vi "DefaultPsTactic.vi"(8 "error in (no error)":errorcluster, 9 "Game in":refnum<class "Game.lvclass">, 10 "Robot":refnum<class "Robot.lvclass">, 11 "DefaultPsTactic in":refnum<class "DefaultPsTactic.lvclass">) -> (0 "error out":errorcluster, 2 "Robot out":refnum<class "Robot.lvclass">, 3 "DefaultPsTactic out":refnum<class "DefaultPsTactic.lvclass">)   [LabVIEW 2018, in "DefaultPsTactic.lvclass"]
uses:
  DefaultPsTactic.lvclass
  C:/Users/anton/Desktop/roboime/PS 2020.1/SSL_AI/Tactic_class/Tactic.lvclass
  Robot_class/Robot.lvclass
  Game_class/Game.lvclass
  Tactic_class/Tactic.lvclass/Tactic.ctl
  TestTactic_class/States.ctl
  Robot_class/tactics.ctl
  Robot_class/Robot.lvclass/Robot.ctl
  Tactic_class/Read Skillbook.vi
  Robot_class/Write tactic.vi
  Skillbook_class/Skillbook.lvclass
  AttackPsSkill_class/AttackPsSkill.lvclass
  DefensePsSkill_class/DefensePsSkill.lvclass
panel:
  out "x .or. y?":bool
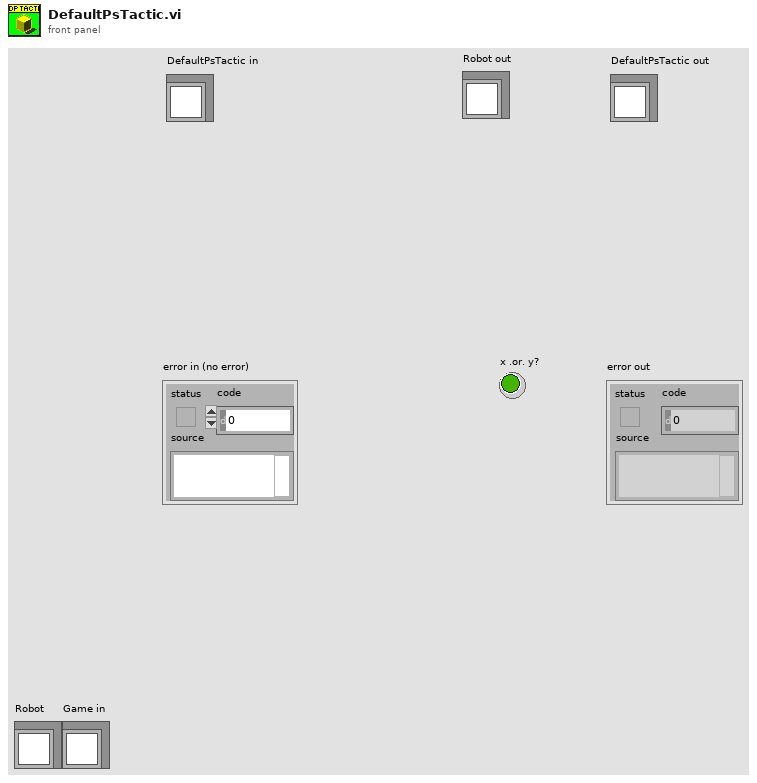
[diagram p1: front panel]
types:
  T1 = typedef "tactics.ctl" = enum16{"PenaltyAttacker", "DefaultPs", "PassObserver", "PenaltyDefense", "Test", "DefendGoal", "Marker", "FollowAttacker", "DefendArea", "Shoot", "AttackerAimGoal", "AttackerBallOutOfField", "AttackerBlock", "AttackerStop", "Duelist", "Halt", "ZigZag", "GoTo", "Timeout", "KickToPassReceiver", "PositionToReceivePass", "PassReceiver", "WaitPass"}
  T2 = typedef "States.ctl" = enum16{"Exit", "AttackPs", "DefensePs"}
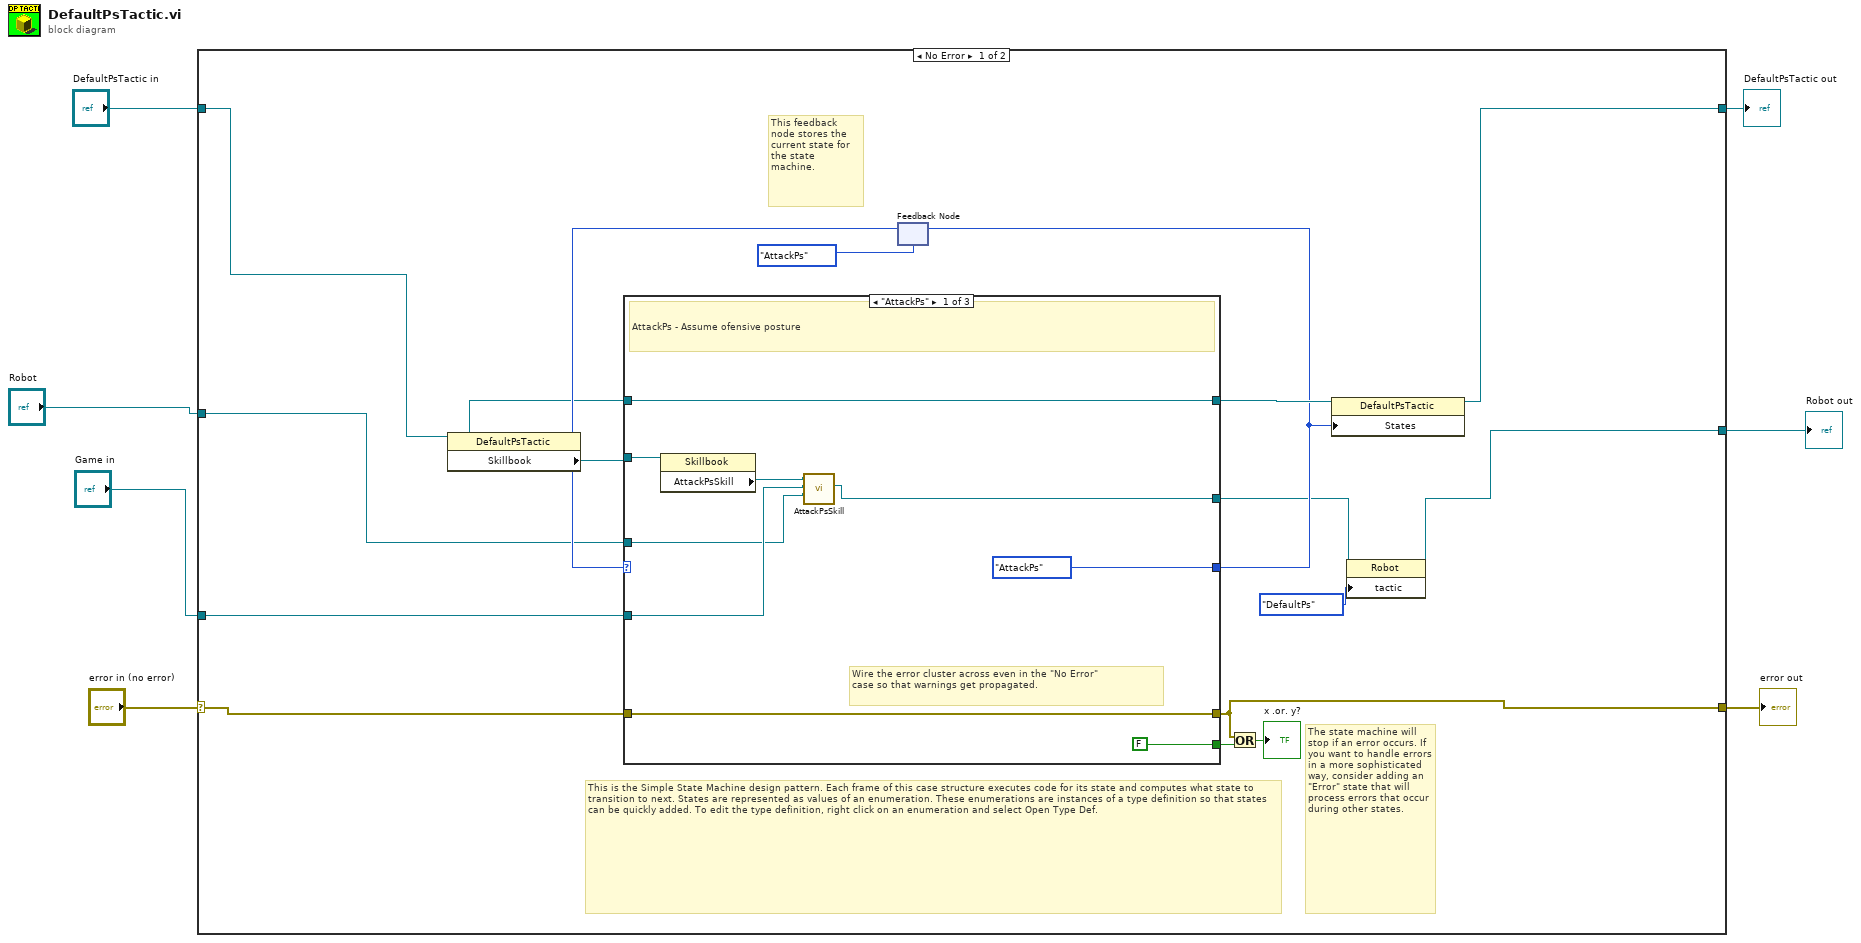
[diagram p0: block diagram]
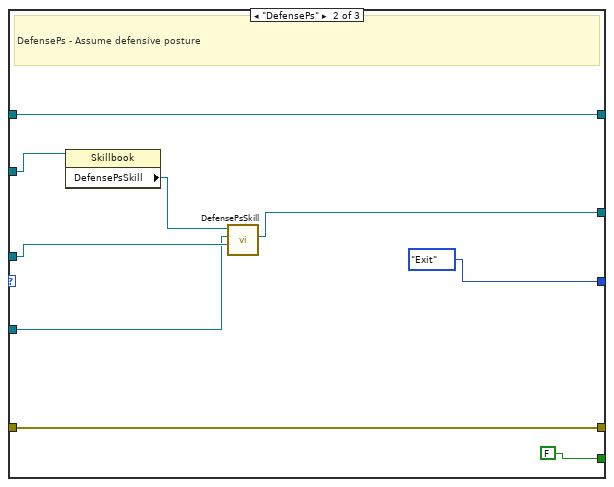
[diagram p2: hidden frame]
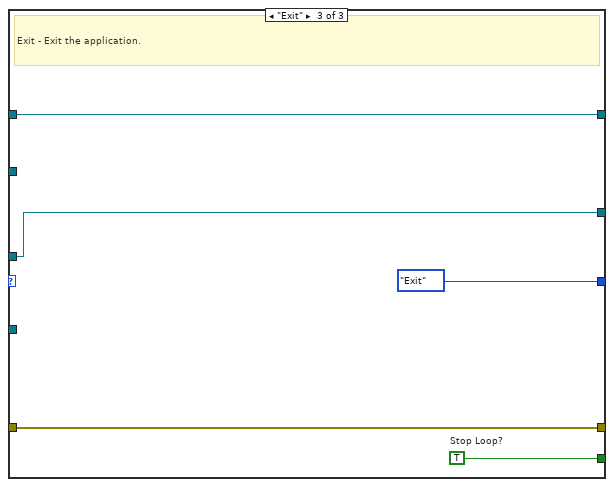
[diagram p3: hidden frame]
diagram:
  n1 = case shown="No Error" "error in (no error)" {
    selector: "error in (no error)" -> [w10 w48]
    tunnel: [w9 w48] -> w6
    tunnel: [w13 w47] -> w4
    tunnel: "DefaultPsTactic in" -> [w14 w47]
    tunnel: "Robot" -> [w12 _]
    tunnel: "Game in" -> [w11 _]
    tunnel: [w8 _] -> w1
    frame No Error {
      # "The state machine will stop if an error occurs. If you want to handle errors in a more sophisticated way, consider adding an \"Error\" state that will process errors that occur during other states."
      # "This feedback node stores the current state for the state machine."
      # "This is the Simple State Machine design pattern. Each frame of this case structure executes code for its state and computes what state to transition to next. States are represented as values of an enumeration. These enumerations are instances of a type definition so that states can be quickly added. To edit the type definition, right click on an enumeration and select Open Type Def."
      # "Wire the error cluster across even in the \"No Error\"\ncase so that warnings get propagated."
      n2 = property class="DefaultPsTactic"(reference=w14) -> ("Skillbook"=w19:refnum<class "Skillbook.lvclass">)  [unwired: 1 in, 2 out]
      n3 = feedback #1(States."AttackPs" ("States")) -> (w21:T2)
      n4 = case shown="\"AttackPs\"" w21 {
        tunnel: [States."AttackPs" ("States") States."Exit" ("States") States."Exit" ("States")] -> w17
        tunnel: [FALSE ("Stop Loop?") FALSE ("Stop Loop?") w46] -> w23
        tunnel: w10 -> [w31 w41 w45]
        tunnel: [w31 w41 w45] -> w9
        tunnel: w19 -> [w29 w40 _]
        tunnel: w12 -> [w25 w37 w43]
        tunnel: [w24 w35 w43] -> w15
        tunnel: [w28 w39 w42] -> w18
        tunnel: w14 -> [w28 w39 w42]
        tunnel: w11 -> [w26 w36 _]
        frame "AttackPs" {
          # "AttackPs - Assume ofensive posture"
          n5 = property class="Skillbook"(reference=w29) -> ("AttackPsSkill"=w27:refnum<class "AttackPsSkill.lvclass">)  [unwired: 1 in, 2 out]
          n6 = call "AttackPsSkill.vi"("Robot"=w25, "Game"=w26, "AttackPsSkill in"=w27) -> ("robot out"=w24:refnum<class "Robot.lvclass">)  [unwired: 6 in, 2 out]
        }
        frame "DefensePs" {
          # "DefensePs - Assume defensive posture"
          n7 = property class="Skillbook"(reference=w40) -> ("DefensePsSkill"=w38:refnum<class "DefensePsSkill.lvclass">)  [unwired: 1 in, 2 out]
          n8 = call "DefensePsSkill.vi"("Robot"=w37, "Game"=w36, "DefensePsSkill in"=w38) -> ("robot out"=w35:refnum<class "Robot.lvclass">)  [unwired: 6 in, 2 out]
        }
        frame "Exit" {
          w46 = TRUE  # Stop Loop?
          # "Exit - Exit the application."
        }
      }
      n9 = feedback-in #1(w17) -> ()
      n10 = Or(x=w9, y=w23) -> (x .or. y?=→"x .or. y?":bool)
      n11 = property class="DefaultPsTactic"(reference=w18, "States"=w17) -> (reference out=w13:refnum<class "DefaultPsTactic.lvclass">)  [unwired: 1 in, 1 out]
      n12 = property class="Robot"(reference=w15, "tactic"=tactics."DefaultPs") -> (reference out=w8:refnum<class "Robot.lvclass">)  [unwired: 1 in, 1 out]
    }
    frame Error {
    }
  }
  "error out" <- w6
  "DefaultPsTactic out" <- w4
  "Robot out" <- w1
